vi "PM-A-myDAQ-read.vi"(8 "error in (no error)":errorcluster, 11 "Refnum in":refnum<k21>) -> (0 "error out":errorcluster, 2 "data":waveform(dbl), 3 "Refnum out":refnum<k21>)   [LabVIEW 2020]
uses:
  <vilib>/DAQmx/read.llb/DAQmx Read (Analog Wfm 1Chan NSamp).vi
  <vilib>/DAQmx/miscellaneous.llb/DAQmx Fill In Error Info.vi
panel:
  out "Waveform Graph":waveform(dbl)(graph)
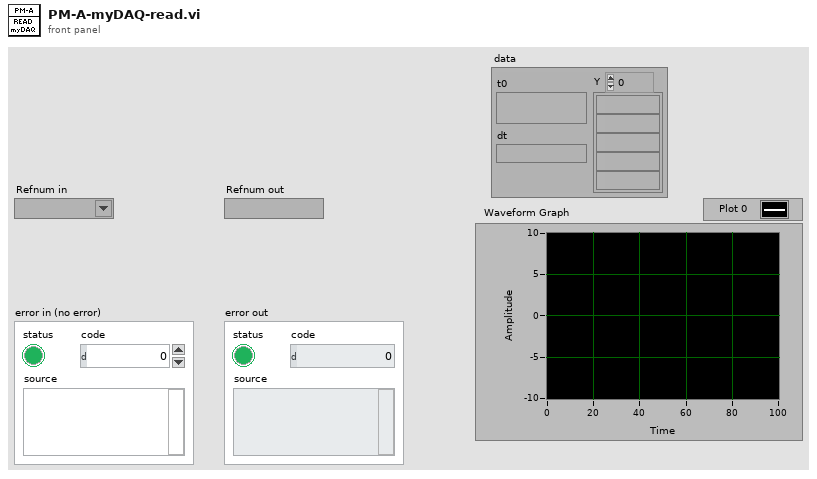
[diagram p1: front panel]
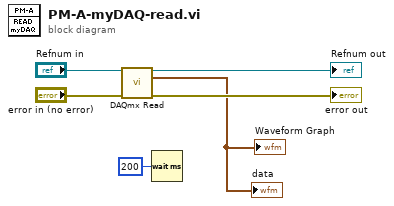
[diagram p0: block diagram]
diagram:
  n1 = call-poly <vilib>:"DAQmx Read.vi"("task/channels in"="Refnum in", "error in"="error in (no error)") -> ("task out"=→"Refnum out":refnum<k21>, "data"=→"data" →"Waveform Graph":waveform(dbl), "error out"=→"error out":errorcluster)  [unwired: 11 in]
  n2 = Wait (ms)(milliseconds to wait=u32 200) -> ()  [unwired: 1 out]
